vi "Pop-up.vi"(4 "Two_btn":bool=TRUE, 6 "IconType":T1=enum."NoIcon", 8 "CancelText":string, 9 "OkText":string, 10 "Text":string, 11 "Title":string) -> (3 "Btn-OK Out":bool)   [LabVIEW 2019]
uses:
  <vilib>/Bytelabs/Message Box/bin/IconType.ctl
  <vilib>/Bytelabs/Message Box/MessageBox.lvlib
panel:
  out "MsgBoxRing-White":u16(ring)
  in  "Btn-Cancel":bool
  in  "Btn-OK":bool
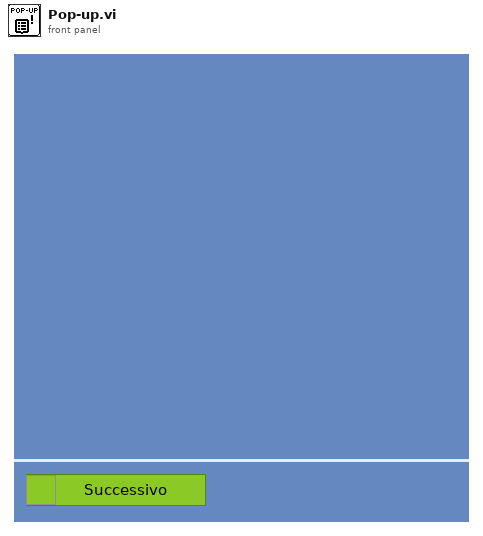
[diagram p1: front panel]
types:
  T1 = typedef "MessageBox.lvlib/IconType.ctl" = enum16{"Error Icon", "NotificationIcon", "QuestionIcon", "InformationIcon", "NoIcon"}
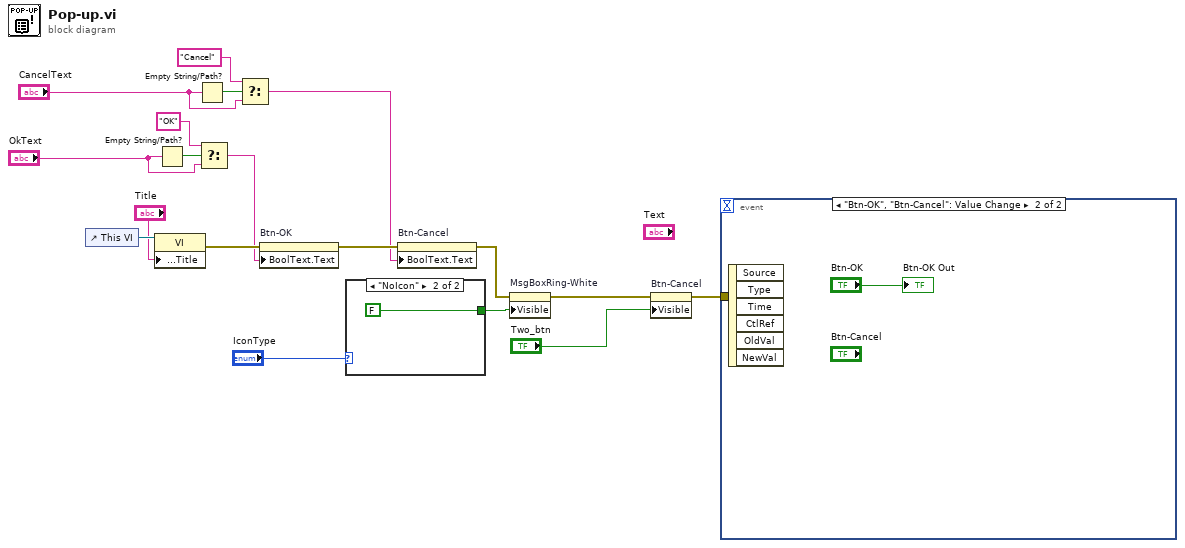
[diagram p0: block diagram]
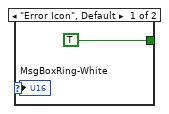
[diagram p2: hidden frame]
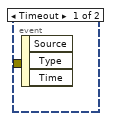
[diagram p3: hidden frame]
diagram:
  n1 = control-ref of="This VI"() -> (w14:refnum<vi>)
  n2 = property class="VI"(reference=w14, "Front Panel.Title"="Title") -> (error out=w13:errorcluster)  [unwired: 1 in, 1 out]
  n3 = Empty String/Path?(string/path="OkText") -> (empty?=w9:bool)
  n4 = Empty String/Path?(string/path="CancelText") -> (empty?=w11:bool)
  n5 = Select(t="OK", s=w9, f="OkText") -> (s? t:f=w7:string)
  n6 = Select(t="Cancel", s=w11, f="CancelText") -> (s? t:f=w6:string)
  n7 = property on="Btn-OK" class="Bool"(error in=w13, "BoolText.Text"=w7) -> (error out=w16:errorcluster)  [unwired: 1 in, 1 out]
  n8 = case shown="\"NoIcon\"" "IconType" {
    selector: "IconType" -> [w19 _]
    tunnel: [TRUE ("Visible") FALSE ("Visible")] -> w17
    frame "Error Icon", Default {
      "MsgBoxRing-White" <- w19
    }
    frame "NoIcon" {
    }
  }
  n9 = property on="Btn-Cancel" class="Bool"(error in=w16, "BoolText.Text"=w6) -> (error out=w15:errorcluster)  [unwired: 1 in, 1 out]
  n10 = property on="MsgBoxRing-White" class="Ring (strict)"(error in=w15, "Visible"=w17) -> (error out=w2:errorcluster)  [unwired: 1 in, 1 out]
  n11 = property on="Btn-Cancel" class="Bool"(error in=w2, "Visible"="Two_btn") -> (error out=w1:errorcluster)  [unwired: 1 in, 1 out]
  n12 = event shown="[1] \"Btn-OK\", \"Btn-Cancel\": Value Change" {
    selector: _ -> [_ _]
    dyn-events: _ -> [_ _]
    timeout: _ -> [_ _]
    tunnel: w1 -> [_ _]
    event Timeout {
      n13 = event-data() -> ()  [unwired: 1 in, 3 out]
    }
    event "Btn-OK", "Btn-Cancel": Value Change {
      n14 = event-data() -> ()  [unwired: 1 in, 6 out]
      "Btn-OK Out" <- "Btn-OK"
    }
  }
